vi "Initialize Plugin.vi"(6 "Resource (blank for prompt)":string, 7 "Instance Name (blank for default)":string, 8 "error in (no error)":errorcluster, 9 "Log Directory":path, 10 "Plugin Path in":path, 11 "Plugin Type":T1) -> (0 "error out":errorcluster, 2 "Failed?":bool, 3 "Generic Controller out":refnum<class "Generic Plugin.lvclass">)   [LabVIEW 2020]
doc: "Initialize a plugin instance based on the information given."
uses:
  Controller/Generic Plugin.lvclass
  Controller/Controller Type.ctl
  <userlib>/Dynamic Reentrant/Dynamic Reentrant.lvlib
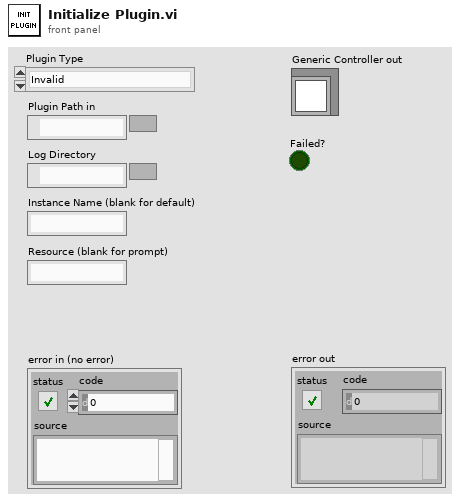
[diagram p1: front panel]
types:
  T1 = typedef "Generic Plugin.lvclass/Controller Type.ctl" = enum16{"Invalid", "Temperature Controller", "Pump Controller", "Generic Optimizer", "LC Parser"}
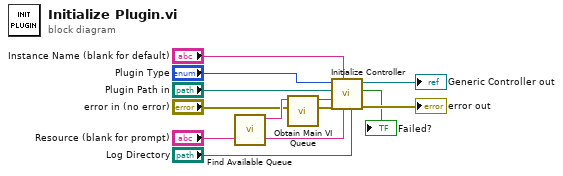
[diagram p0: block diagram]
diagram:
  n1 = call "Find Available Queue.vi"() -> ("String"=w8:string)  [unwired: 11 in]
  n2 = call <userlib>:"Obtain Main VI Queue.vi"("error in (no error)"="error in (no error)", "Name (Main VI)"=w8) -> ("error out"=w10:errorcluster, "queue out"=w9:refnum<queue>)  [unwired: 8 in]
  n3 = call "Initialize Controller.vi"("Log Directory"="Log Directory", "Resource"="Resource (blank for prompt)", "Instance Name"="Instance Name (blank for default)", "error in (no error)"=w10, "Receiving Queue"=w9, "Control Panel Path"="Plugin Path in", "Controller Type"="Plugin Type") -> ("error out"=→"error out":errorcluster, "Failed?"=→"Failed?":bool, "Generic Controller out"=→"Generic Controller out":refnum<class "Generic Plugin.lvclass">)  [unwired: 2 in]
